vi "Read_imaging_cfg.vi"(8 "error in (no error)":errorcluster, 10 "Config.ini Path":path) -> (0 "error out":errorcluster, 3 "System Parameters":T1={"Optical Parameters"={"Obj. Focal Length [mm]"=0.0, "Scan Lens EFL[mm]"=0.0, "Tube Lens EFL[mm]"=0.0, "Galvo V Range (+/-)"=0.0, "Galvo Max Half Angle [Deg]"=0.0, "Max Galvo Range[%]"=0.0}, "Vibratome"={"Pre Cut Dwell [s]"=0.0, "Blade Frequency [RPM]"=0, "Slice Speed [mm/s]"=0.0, "Post Cut Dwell [s]"=0.0, "Ramp Time [s]"=0.0, "Start X [mm]"=0.0, "Start Y [mm]"=0.0, "Slice Length [mm]"=0.0, "Slice Axis"=enum."Y Axis", "Controller VISA Ref"="COM4", "Blade Frequency [Hz]"=0, "Analog Out Channel"="GalvoCtrl/ao0,GalvoCtrl/ao1", "Pixel Clock Source"="/GalvoCtrl/PFI0", "Vib version"=enum."Vibratome1"}, "Table Stages"={"X Stage"={"Position"=0.0, "Is.Enabled?"=FALSE, "Is.Connected?"=FALSE, "Device SN"="45876539", "AccelerationMaximum"=0.0, "VelocityMaximum"=0.0, "Acceleration"=0.0, "Velocity"=0.0, "waitTimeout (ms)"=0, "Model"=enum."None", "Is.Homed?"=FALSE, "MOVE"=FALSE}, "Y Stage"={"Position"=0.0, "Is.Enabled?"=FALSE, "Is.Connected?"=FALSE, "Device SN"="45876539", "AccelerationMaximum"=0.0, "VelocityMaximum"=0.0, "Acceleration"=0.0, "Velocity"=0.0, "waitTimeout (ms)"=0, "Model"=enum."None", "Is.Homed?"=FALSE, "MOVE"=FALSE}, "Z Stage"={"Position"=0.0, "Is.Enabled?"=FALSE, "Is.Connected?"=FALSE, "Device SN"="45876539", "AccelerationMaximum"=0.0, "VelocityMaximum"=0.0, "Acceleration"=0.0, "Velocity"=0.0, "waitTimeout (ms)"=0, "Model"=enum."None", "Is.Homed?"=FALSE, "MOVE"=FALSE}, "Attenuator"={"Position"=0.0, "Is.Enabled?"=FALSE, "Is.Connected?"=FALSE, "Device SN"="45876539", "AccelerationMaximum"=0.0, "VelocityMaximum"=0.0, "Acceleration"=0.0, "Velocity"=0.0, "waitTimeout (ms)"=0, "Model"=enum."None", "Is.Homed?"=FALSE, "MOVE"=FALSE}}, "Imaging Parameter"={"Raster Scan Direction"=enum."Bi Directional", "Pixel Dwell Time [Clock Cycles]"=1, "Flyback Time [Clock Cycles]"=200, "XY Center [um]"={"X"=1.0, "Y"=1.0}, "Pixel Step Size [um] X"=2.5, "XY Image Size"=enum."2048 x 2048", "Custom"=FALSE, "Custom Size"={"X"=1, "Y"=1}, "Line Averages"=1, "Pixel Step Size [um] Y"=0.0}, "Galvo HW Parameters"={"Analog Out Channel"="GalvoCtrl/ao0,GalvoCtrl/ao1", "Min Voltage"=-10.0, "Max Voltage"=10.0, "Pixel Clock Source"="/GalvoCtrl/PFI0", "Sample Rate"=1000.0, "Line Clock Out Ch"="GalvoCtrl/port0/line0", "2P ready check"="GalvoCtrl/port0/line0"}, "Alazar parameters"={"Trigger Settings"={"General Trigger Settings"={"Trigger Operation"=0, "Coupling ID"=2, "Range ID"=2, "Delay"=0, "Timeout Ticks"=0, "Mode"=1, "Parameter"=1}, "Trigger Engine 1"={"Trigger Engine"=0, "Source"=2, "Slope"=1, "Level"=140}, "Trigger Engine 2"={"Trigger Engine"=1000, "Source"=4294967295, "Slope"=1, "Level"=2048}}, "Device ID"={"System ID"=1, "Board ID"=1}, "Ch A Input Control"={"Channel"=1, "Coupling"=2, "Range"=10, "Impedance"=2}, "Ch B Input Control"={"Channel"=2, "Coupling"=2, "Range"=10, "Impedance"=2}, "Acq Settings"={"Record Length"=1440, "Offset"=0, "Records Per Buffer"=2048, "Records Count (Records/Acq)"=2147483647, "Window Type"=1, "Footer"=0, "Samples per record"=2048, "Output Format"=257}, "Capture Clock"={"Sample Rate"=100, "Decimation"=0, "Source"=2, "Edge"=0}}, "Mosaic Paramter"={"X Axis"={"Start [mm]"=0.0, "Steps [pts]"=0.0, "End [mm]"=0.0}, "Y Axis"={"Start [mm]"=0.0, "Steps [pts]"=0.0, "End [mm]"=0.0}, "Scan Pattern"=enum."Uni-directional", "Overlap Options"={"Overlap Type"=enum."No Overlap", "Percent Overlap"=0, "Justify"=enum."Start"}}, "Manual Controls"={"Data Path"=path "", "Save parameters"={"start pixel"=45, "#pixels to save"=100}, "Acquisition mode"=enum."Alazar FFT", "PSOCT Channel"=1, "Save data?"=FALSE, "AIP rotation angle"=3.0, "Pause acquisition?"=FALSE, "Outgoing Mail Server (SMTP)"="smtp.gmail.com", "Email"="", "Password"="", "Carrier 1"=enum."Sprint", "phone number 1"="", "Subject"="", "Message"="", "Carrier 2"=enum."Sprint", "phone number 2"="", "Check boundary?"=FALSE, "Threshold"=0.0, "Outputs for GPU FFT"=enum."Amp + Phase diff", "Slice# init"=1}, "Z stage setting"={"first cut height(mm)"=45.85, "slice thickness[um]"=[], "#cycles"=111, "image thickness(um)"=[], "First image height(mm)"=2.1, "Pause?"=[], "Z0"=0.0, "fixed Z0?"=FALSE, "Save PSOCT?"=[]}, "Attenuator"={"Power after Objective (recalibrate every 6 month)"=[]}} {"Manual Controls"."PSOCT Channel" items=["A"=1, "B"=2, "A + B"=3, "C"=4, "A + C"=5, "A + B"=6, "D"=8, "A + D"=9, "B + D"=10, "C + D"=12, "A + B + C + D"=15]; "Alazar parameters"."Capture Clock"."Edge" items=["Rising", "Falling"]; "Alazar parameters"."Capture Clock"."Source" items=["Internal"=1, "Fast External"=2, "Medium External"=3, "Slow External"=4, "External AC"=5, "External DC"=6, "External 10MHz"=7]; "Alazar parameters"."Acq Settings"."Output Format" items=["Float Log"=11, "Float Amp"=10, "U16_LOG"=1, "U16_AMP2"=257, "Real"=3, "Imag"=4]; "Alazar parameters"."Acq Settings"."Footer" items=["FOOTER_NONE", "FOOTER_NPT"]; "Alazar parameters"."Acq Settings"."Window Type" items=["DSP_WINDOW_NONE", "DSP_WINDOW_HANNING", "DSP_WINDOW_HAMMING", "DSP_WINDOW_BLACKMAN", "DSP_WINDOW_BLACKMAN_HARRIS", "DSP_WINDOW_BARTLETT"]; "Alazar parameters"."Ch B Input Control"."Channel" items=["A"=1, "B"=2, "C"=4, "D"=8]; "Alazar parameters"."Ch B Input Control"."Coupling" items=["AC"=1, "DC"=2]; "Alazar parameters"."Ch B Input Control"."Range" items=["20 mV"=1, "40 mV"=2, "50 mV"=3, "80 mV"=4, "100 mV"=5, "200 mV"=6, "400 mV"=7, "500 mV"=8, "800 mV"=9, "1 V"=10, "1.25 V"=33, "2 V"=11, "4 V"=12, "5 V"=13, "8 V"=14, "10 V"=15, "20 V"=16]; "Alazar parameters"."Ch B Input Control"."Impedance" items=["1 MOhm"=1, "50 Ohm"=2, ""=0]; "Alazar parameters"."Ch A Input Control"."Channel" items=["A"=1, "B"=2, "C"=4, "D"=8]; "Alazar parameters"."Ch A Input Control"."Coupling" items=["AC"=1, "DC"=2]; "Alazar parameters"."Ch A Input Control"."Range" items=["20 mV"=1, "40 mV"=2, "50 mV"=3, "80 mV"=4, "100 mV"=5, "200 mV"=6, "400 mV"=7, "500 mV"=8, "800 mV"=9, "1 V"=10, "1.25 V"=33, "2 V"=11, "4 V"=12, "5 V"=13, "8 V"=14, "10 V"=15, "20 V"=16]; "Alazar parameters"."Ch A Input Control"."Impedance" items=["1 MOhm"=1, "50 Ohm"=2, ""=0]; "Alazar parameters"."Trigger Settings"."General Trigger Settings"."Trigger Operation" items=["J", "K", "J OR K", "J AND K", "J XOR K", "J AND NOT K", "NOT J AND K"]; "Alazar parameters"."Trigger Settings"."General Trigger Settings"."Coupling ID" items=["AC"=1, "DC"=2]; "Alazar parameters"."Trigger Settings"."General Trigger Settings"."Range ID" items=["5 V", "1 V", "TTL"]; "Alazar parameters"."Trigger Settings"."Trigger Engine 1"."Trigger Engine" items=["J", "K"]; "Alazar parameters"."Trigger Settings"."Trigger Engine 1"."Source" items=["A", "B", "External", "Disable", "C", "D"]; "Alazar parameters"."Trigger Settings"."Trigger Engine 1"."Slope" items=["Positive"=1, "Negative"=2]; "Alazar parameters"."Trigger Settings"."Trigger Engine 2"."Trigger Engine" items=["J", "K"]; "Alazar parameters"."Trigger Settings"."Trigger Engine 2"."Source" items=["A", "B", "External", "Disable", "C", "D"]; "Alazar parameters"."Trigger Settings"."Trigger Engine 2"."Slope" items=["Positive"=1, "Negative"=2]; "Imaging Parameter"."Pixel Step Size [um] Y" min=0.0 max=100.0 step=0.01; "Imaging Parameter"."Line Averages" min=1 max=30 step=1; "Imaging Parameter"."Flyback Time [Clock Cycles]" max=10 step=1; "Imaging Parameter"."Pixel Step Size [um] X" min=0.0 max=100.0 step=0.01; "Imaging Parameter"."Custom Size"."Y" min=1 max=30 step=1; "Imaging Parameter"."Custom Size"."X" min=1 max=30 step=1; "Imaging Parameter"."XY Center [um]"."Y" min=1.0 max=30.0 step=1.0; "Imaging Parameter"."XY Center [um]"."X" min=1.0 max=30.0 step=1.0; "Imaging Parameter"."Pixel Dwell Time [Clock Cycles]" max=10 step=1})   [LabVIEW 2018]
uses:
  Controls/System Parameters.ctl
  Controls/Optical Parameters.ctl
  Controls/Vibratome Parameters.ctl
  type defines/vibratome.ctl
  Controls/Translation Stage Parameters.ctl
  Hardware Mfg/Thorlabs Translation Stages/Controls/Translation Stage Cluster.ctl
  Controls/Translation Stage Types.ctl
  Controls/Imaging Parameters.ctl
  Controls/Scan Direction.ctl
  type defines/Alazar parameters.ctl
  Hardware Mfg/AlazarTech SDK/Controls/General Trigger Settings.ctl
  Hardware Mfg/AlazarTech SDK/Controls/Trigger Engine Controls.ctl
  Hardware Mfg/AlazarTech SDK/Controls/Alazar Device ID.ctl
  Hardware Mfg/AlazarTech SDK/Controls/Channel Input Controls.ctl
  Hardware Mfg/AlazarTech SDK/Controls/Alazar Acquisition Settings.ctl
  Hardware Mfg/AlazarTech SDK/Controls/Clock Controls.ctl
  type defines/Mosaic Parameter.ctl
  type defines/Manual Controls.ctl
  type defines/FFT parameters.ctl
  type defines/FFT mode.ctl
  type defines/GPU FFT outputs.ctl
  type defines/Vibratome Param.ctl
  type defines/attenuator.ctl
  <vilib>/Utility/config.llb/NI_LVConfig.lvlib
panel:
  # "X"
  # "X"
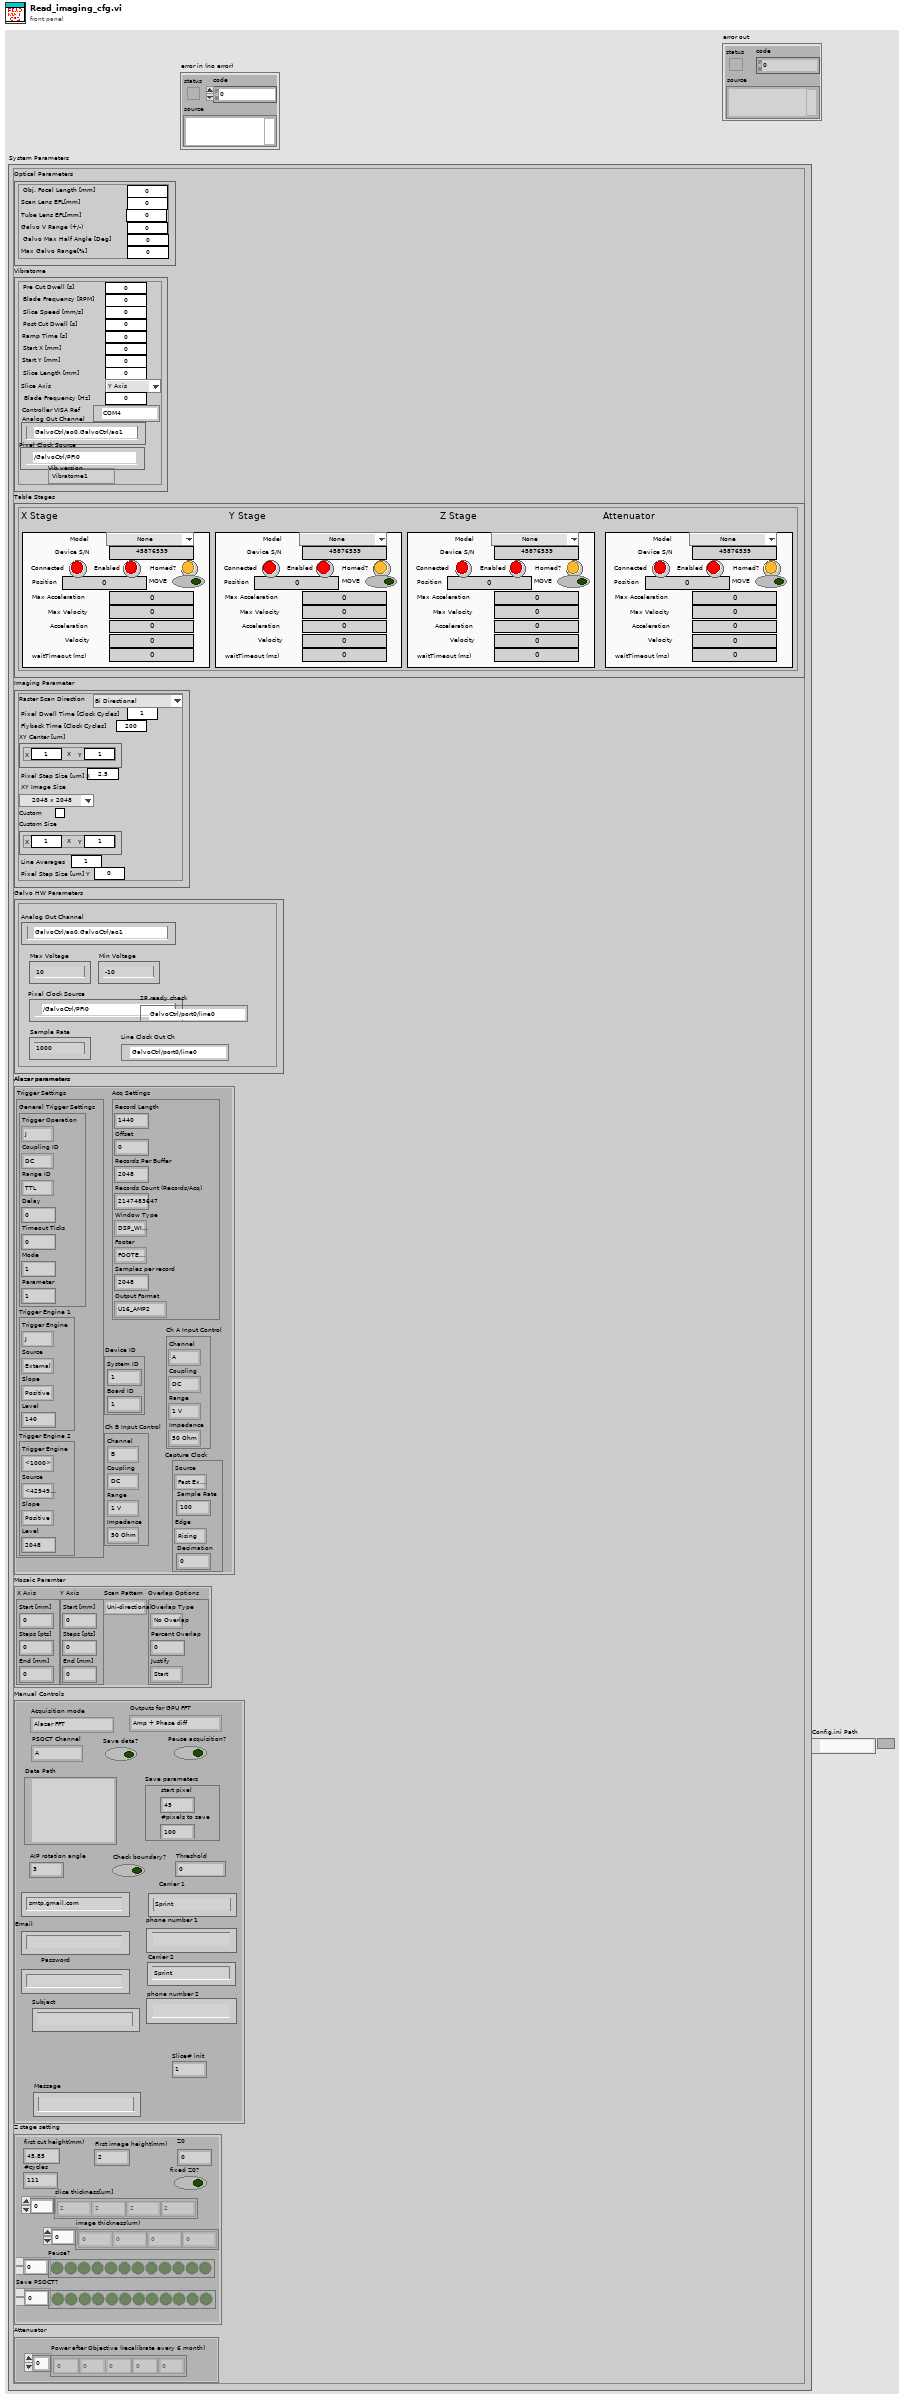
[diagram p1: front panel]
types:
  T1 = typedef "System Parameters.ctl" = cluster{"Optical Parameters":T2, "Vibratome":T3, "Table Stages":T5, "Imaging Parameter":T8, "Galvo HW Parameters":cluster{"Analog Out Channel":tag, "Min Voltage":dbl, "Max Voltage":dbl, "Pixel Clock Source":tag, "Sample Rate":dbl, "Line Clock Out Ch":tag, "2P ready check":tag}, "Alazar parameters":T10, "Mosaic Paramter":T17, "Manual Controls":T18, "Z stage setting":T22, "Attenuator":T23}
  T2 = typedef "Optical Parameters.ctl" = cluster{"Obj. Focal Length [mm]":dbl, "Scan Lens EFL[mm]":dbl, "Tube Lens EFL[mm]":dbl, "Galvo V Range (+/-)":dbl, "Galvo Max Half Angle [Deg]":dbl, "Max Galvo Range[%]":dbl}
  T3 = typedef "Vibratome Parameters.ctl" = cluster{"Pre Cut Dwell [s]":dbl, "Blade Frequency [RPM]":u16, "Slice Speed [mm/s]":dbl, "Post Cut Dwell [s]":dbl, "Ramp Time [s]":dbl, "Start X [mm]":dbl, "Start Y [mm]":dbl, "Slice Length [mm]":dbl, "Slice Axis":enum16{"X Axis", "Y Axis", "Z Axis"}, "Controller VISA Ref":refnum<visa-resource-name>, "Blade Frequency [Hz]":u16, "Analog Out Channel":tag, "Pixel Clock Source":tag, "Vib version":T4}
  T4 = typedef "vibratome.ctl" = enum16{"Vibratome1", "Vibratome3"}
  T5 = typedef "Translation Stage Parameters.ctl" = cluster{"X Stage":T6, "Y Stage":T6, "Z Stage":T6, "Attenuator":T6}
  T6 = typedef "Translation Stage Cluster.ctl" = cluster{"Position":dbl, "Is.Enabled?":bool, "Is.Connected?":bool, "Device SN":string, "AccelerationMaximum":dbl, "VelocityMaximum":dbl, "Acceleration":dbl, "Velocity":dbl, "waitTimeout (ms)":i32, "Model":T7, "Is.Homed?":bool, "MOVE":bool}
  T7 = typedef "Translation Stage Types.ctl" = enum16{"None", "Thorlabs LTS", "Thorlabs MLJ"}
  T8 = typedef "Imaging Parameters.ctl" = cluster{"Raster Scan Direction":T9, "Pixel Dwell Time [Clock Cycles]":u16, "Flyback Time [Clock Cycles]":u16, "XY Center [um]":cluster{"X":dbl, "Y":dbl}, "Pixel Step Size [um] X":dbl, "XY Image Size":enum16{"32 x 32", "64 x 64", "128 x 128", "256 x 256", "512 x 512", "1024 x 1024", "2048 x 2048"}, "Custom":bool, "Custom Size":cluster{"X":u16, "Y":u16}, "Line Averages":u16, "Pixel Step Size [um] Y":dbl}
  T9 = typedef "Scan Direction.ctl" = enum16{"Uni Directional", "Bi Directional", "None"}
  T10 = typedef "Alazar parameters.ctl" = cluster{"Trigger Settings":cluster{"General Trigger Settings":T11, "Trigger Engine 1":T12, "Trigger Engine 2":T12}, "Device ID":T13, "Ch A Input Control":T14, "Ch B Input Control":T14, "Acq Settings":T15, "Capture Clock":T16}
  T11 = typedef "General Trigger Settings.ctl" = cluster{"Trigger Operation":u32, "Coupling ID":u32, "Range ID":u32, "Delay":u32, "Timeout Ticks":u32, "Mode":u32, "Parameter":u32}
  T12 = typedef "Trigger Engine Controls.ctl" = cluster{"Trigger Engine":u32, "Source":u32, "Slope":u32, "Level":u32}
  T13 = typedef "Alazar Device ID.ctl" = cluster{"System ID":u32, "Board ID":u32}
  T14 = typedef "Channel Input Controls.ctl" = cluster{"Channel":u8, "Coupling":u32, "Range":u32, "Impedance":u32}
  T15 = typedef "Alazar Acquisition Settings.ctl" = cluster{"Record Length":u32, "Offset":u32, "Records Per Buffer":u32, "Records Count (Records/Acq)":u32, "Window Type":u32, "Footer":u32, "Samples per record":u32, "Output Format":u32}
  T16 = typedef "Clock Controls.ctl" = cluster{"Sample Rate":u32, "Decimation":u32, "Source":u32, "Edge":u32}
  T17 = typedef "Mosaic Parameter.ctl" = cluster{"X Axis":cluster{"Start [mm]":dbl, "Steps [pts]":dbl, "End [mm]":dbl}, "Y Axis":cluster{"Start [mm]":dbl, "Steps [pts]":dbl, "End [mm]":dbl}, "Scan Pattern":enum16{"Uni-directional", "Bi-Directional", "Spiral Out", "Spiral In"}, "Overlap Options":cluster{"Overlap Type":enum16{"No Overlap", "X Only", "Y Only", "X and Y"}, "Percent Overlap":u8, "Justify":enum16{"Start", "Center", "End"}}}
  T18 = typedef "Manual Controls.ctl" = cluster{"Data Path":path, "Save parameters":T19, "Acquisition mode":T20, "PSOCT Channel":u32, "Save data?":bool, "AIP rotation angle":dbl, "Pause acquisition?":bool, "Outgoing Mail Server (SMTP)":string, "Email":string, "Password":string, "Carrier 1":enum16{"T-Mobile", "AT&T", "Verizon", "Sprint"}, "phone number 1":string, "Subject":string, "Message":string, "Carrier 2":enum16{"T-Mobile", "AT&T", "Verizon", "Sprint"}, "phone number 2":string, "Check boundary?":bool, "Threshold":sgl, "Outputs for GPU FFT":T21, "Slice# init":i32}
  T19 = typedef "FFT parameters.ctl" = cluster{"start pixel":i32, "#pixels to save":i32}
  T20 = typedef "FFT mode.ctl" = enum16{"ThorOCT B line", "ThorOCT Spectral", "ThorOCT FFT", "Alazar B line", "Alazar FFT", "GPU FFT", "Alazar Spectral", "Simulation", "auto adjust focus", "Save all"}
  T21 = typedef "GPU FFT outputs.ctl" = enum16{"Amp + Phase diff", "Amp + Phase", "Amp only"}
  T22 = typedef "Vibratome Param.ctl" = cluster{"first cut height(mm)":dbl, "slice thickness[um]":u32[], "#cycles":u16, "image thickness(um)":u32[], "First image height(mm)":dbl, "Pause?":bool[], "Z0":dbl, "fixed Z0?":bool, "Save PSOCT?":bool[]}
  T23 = typedef "attenuator.ctl" = cluster{"Power after Objective (recalibrate every 6 month)":dbl[]}
  T24 = typedef "NI_LVConfig.lvlib/Config Data RefNum.ctl" = refnum<k1>
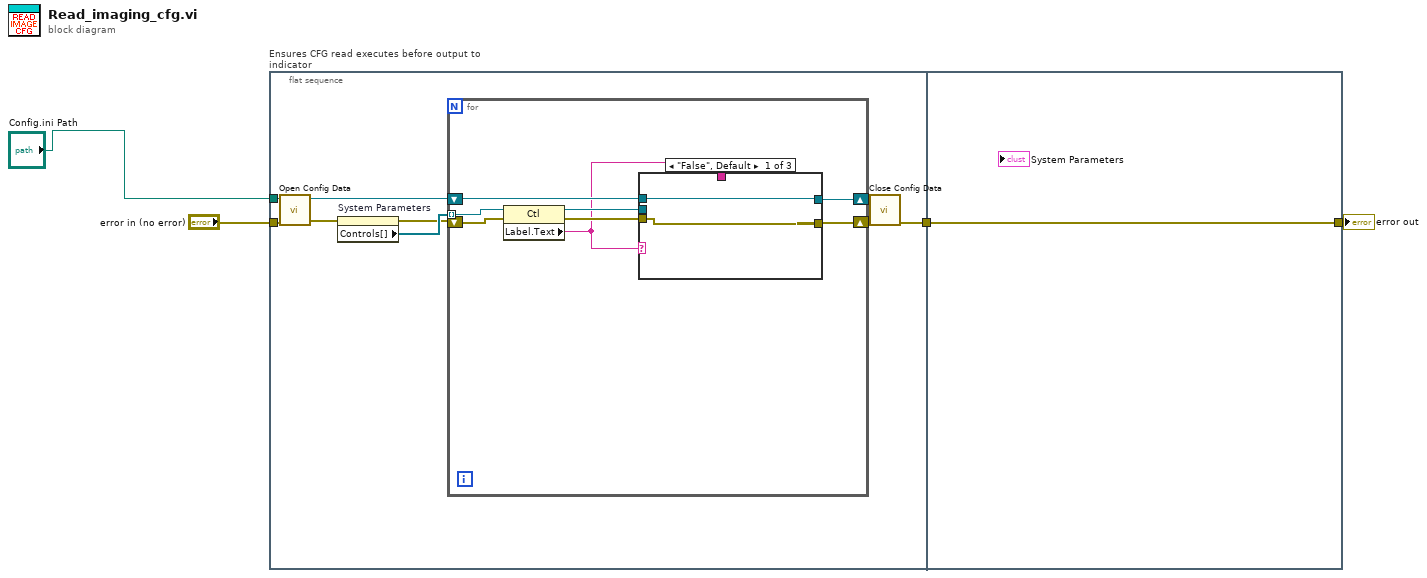
[diagram p0: block diagram]
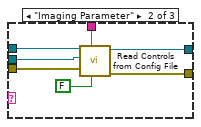
[diagram p2: hidden frame]
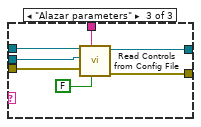
[diagram p3: hidden frame]
diagram:
  n1 = flat-sequence "Ensures CFG read executes before output to indicator" {
    tunnel: "error in (no error)" -> [w13]
    tunnel: "Config.ini Path" -> [w11]
    tunnel: [w12] -> w4
    tunnel: [w38] -> w2
    tunnel: w4 -> [w38]
    frame #0 {
      n2 = call <vilib>:"Open Config Data.vi"("error in (no error)"=w13, "configuration file path"=w11) -> ("error out"=w5:errorcluster, "refnum"=w8:T24)  [unwired: 7 in, 1 out]
      n3 = property on="System Parameters" class="Clust (strict)"(error in=w5) -> (error out=w6:errorcluster, "Controls[]"=w10:refnum<vi>[])  [unwired: 1 in, 1 out]
      n4 = for {
        tunnel: w10 -> [w21] mode=indexing
        shift-right: [w18] -> w9
        shift-left: w6 -> [w20]
        shift-right: [w15] -> w7
        shift-left: w8 -> [w17]
        n5 = property class="Ctl"(reference=w21, error in=w20) -> (reference out=w16:refnum<vi>, error out=w19:errorcluster, "Label.Text"=w14:string)
        n6 = case shown="\"False\", Default" w14 {
          tunnel: w19 -> [w23 w29 w36]
          tunnel: [w23 w28 w35] -> w18
          tunnel: w17 -> [w22 w27 w34]
          tunnel: w16 -> [_ w26 w33]
          tunnel: w14 -> [_ w25 w32]
          tunnel: [w22 w24 w31] -> w15
          frame "False", Default {
          }
          frame "Imaging Parameter" {
            n7 = call "Read Controls from Config File.vi"("Child?"=FALSE, "section"=w25, "Error In"=w29, "Ctl Refnum"=w26, "refnum"=w27) -> ("Error Out"=w28:errorcluster, "refnum out"=w24:T24)  [unwired: 5 in]
          }
          frame "Alazar parameters" {
            n8 = call "Read Controls from Config File.vi"("Child?"=FALSE, "section"=w32, "Error In"=w36, "Ctl Refnum"=w33, "refnum"=w34) -> ("Error Out"=w35:errorcluster, "refnum out"=w31:T24)  [unwired: 5 in]
          }
        }
      }
      n9 = call <vilib>:"Close Config Data.vi"("error in (no error)"=w9, "refnum"=w7) -> ("error out"=w12:errorcluster)  [unwired: 8 in, 1 out]
    }
    frame #1 {
    }
  }
  "error out" <- w2
